vi "Split Inverted Commas.vi"(11 "String in":string) -> (3 "String out":string)   [LabVIEW 2013]
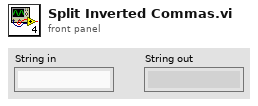
[diagram p1: front panel]
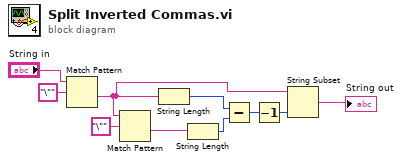
[diagram p0: block diagram]
diagram:
  n1 = Match Pattern(string="String in", regular expression="\"") -> (after substring=w8:string)  [unwired: 1 in, 3 out]
  n2 = Match Pattern(string=w8, regular expression="\"") -> (after substring=w3:string)  [unwired: 1 in, 3 out]
  n3 = String Length(string=w8) -> (length=w5:i32)
  n4 = String Length(string=w3) -> (length=w4:i32)
  n5 = Subtract(x=w5, y=w4) -> (x-y=w6:i32)
  n6 = Decrement(x=w6) -> (x-1=w9:i32)
  n7 = String Subset(string=w8, length (rest)=w9) -> (substring=→"String out":string)  [unwired: 1 in]
